vi "Insert Value (Nested String).vi"(7 "key":string[](array[string]), 8 "error in (no error)":errorcluster, 10 "JSON Data in":string, 11 "JSON Value in":refnum<class "JSON Value.lvclass">) -> (0 "error out":errorcluster, 1 "replaced":bool, 3 "JSON Value out":refnum<class "JSON Value.lvclass">)   [LabVIEW 2016, in "JSON Value.lvclass"]
uses:
  JSON Value.lvclass
  New JSON Value/New JSON String.vi
  Insert Value (Single).vi
  Array/Replace Array Subset/Replace Array Subset (Single).vi
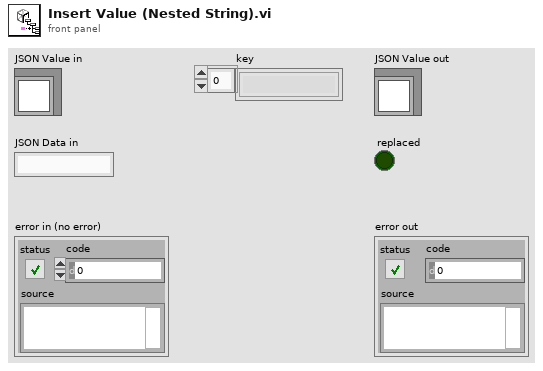
[diagram p1: front panel]
types:
  T1 = typedef "JSON Value.lvclass/JSON Types.ctl" = enum16{"String", "Numeric", "Boolean", "NULL", "Object", "Array"}
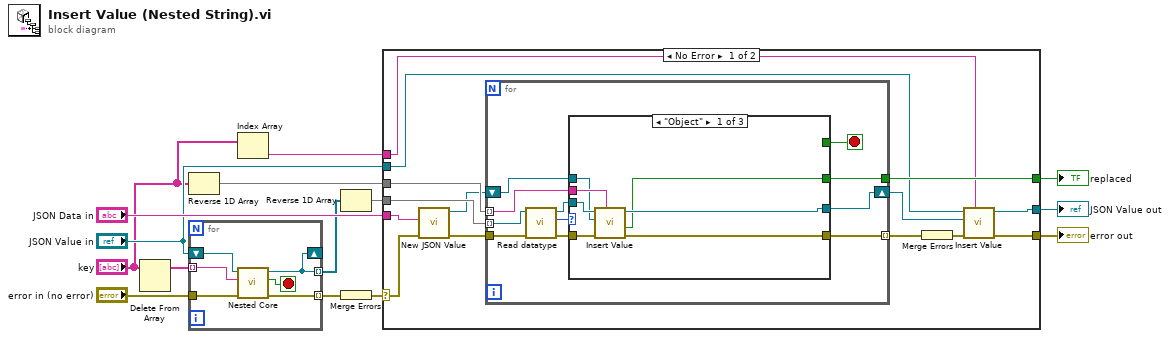
[diagram p0: block diagram]
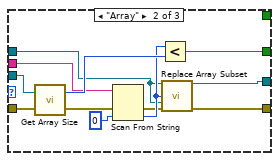
[diagram p2: hidden frame]
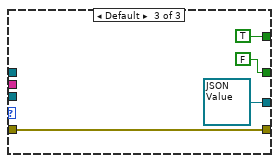
[diagram p3: hidden frame]
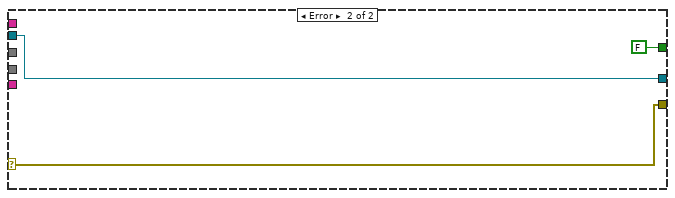
[diagram p4: hidden frame]
diagram:
  n1 = Delete From Array(array="key") -> (array with subset deleted=w10:string[])  [unwired: 2 in, 1 out]
  n2 = Reverse 1D Array(array="key") -> (reversed array=w11:string[])
  n3 = for {
    tunnel: w10 -> [w20] mode=indexing
    shift-right: [w15] -> _
    shift-left: "JSON Value in" -> [w19]
    tunnel: "error in (no error)" -> [w18]
    tunnel: [w17] -> w7 mode=indexing
    tunnel: [w15] -> w8 mode=indexing
    stop <- w16 stop-if-true
    n4 = call "Nested Core.vi"("error in (no error)"=w18, "key"=w20, "JSON Value in"=w19) -> ("error out"=w17:errorcluster, "stop?"=w16:bool, "JSON Value out"=w15:refnum<class "JSON Value.lvclass">)  [unwired: 6 in]
  }
  n5 = Index Array(array="key") -> (element=w1:string)  [unwired: 1 in]
  n6 = Reverse 1D Array(array=w8) -> (reversed array=w12:refnum<class "JSON Value.lvclass">[])
  n7 = Merge Errors(w7) -> (w9:errorcluster)
  n8 = case shown="No Error" w9 {
    selector: w9 -> [w22 w69]
    tunnel: [w34 FALSE ("replaced")] -> w14
    tunnel: "JSON Data in" -> [w24 _]
    tunnel: w12 -> [w33 _]
    tunnel: w11 -> [w32 _]
    tunnel: [w28 w71] -> w4
    tunnel: "JSON Value in" -> [w30 w71]
    tunnel: [w26 w69] -> w3
    tunnel: w1 -> [w25 _]
    frame No Error {
      n9 = call-poly "New JSON Value.vi"("error in (no error)"=w22, "value"=w24) -> ("error out"=w21:errorcluster, "JSON Value out"=w23:refnum<class "JSON Value.lvclass">)  [unwired: 8 in]
      n10 = for {
        tunnel: w32 -> [w37] mode=indexing
        tunnel: w21 -> [w43]
        tunnel: [w42] -> w31 mode=indexing
        tunnel: [w39] -> w34
        tunnel: w33 -> [w38] mode=indexing
        shift-right: [w36] -> w29
        shift-left: w23 -> [w35]
        stop <- w40 stop-if-true
        n11 = call "Read datatype.vi"("error in (no error)"=w43, "JSON Datatype in"=w38) -> ("error out"=w41:errorcluster, "datatype"=w44:T1, "JSON Datatype out"=w45:refnum<class "JSON Value.lvclass">)  [unwired: 7 in]
        n12 = case shown="\"Object\"" w44 {
          tunnel: w37 -> [w49 w61 _]
          tunnel: [w51 w59 refnum<class "JSON Value.lvclass"> refnum ("JSON Array")] -> w36
          tunnel: w45 -> [w48 w60 _]
          tunnel: [w52 w53 w67] -> w42
          tunnel: w41 -> [w47 w56 w67]
          tunnel: [_ _ TRUE] -> w40
          tunnel: [w50 w62 FALSE] -> w39
          tunnel: w35 -> [w46 w57 _]
          frame "Object" {
            n13 = call-poly "Insert Value.vi"("key"=w49, "error in (no error)"=w47, 10:"JSON Value in"=w46, 11:"JSON Value in"=w48) -> ("error out"=w52:errorcluster, "replaced"=w50:bool, "JSON Value out"=w51:refnum<class "JSON Value.lvclass">)  [unwired: 5 in]
          }
          frame "Array" {
            n14 = call "Get Array Size.vi"("error in (no error)"=w56, "JSON Value in"=w60) -> ("error out"=w55:errorcluster, "size(s)"=w63:i32)
            n15 = Scan From String(input string=w61, error in=w55, default 1=0 ("index")) -> (error out=w54:errorcluster, output 1=w58:i32)  [unwired: 2 in, 2 out]
            n16 = Less?(x=w58, y=w63) -> (x < y?=w62:bool)
            n17 = call-poly "Replace Array Subset.vi"("JSON Array"=w57, "index"=w58, "new element/subarray"=w57, "error in"=w54) -> ("output JSON Array"=w59:refnum<class "JSON Value.lvclass">, "error out"=w53:errorcluster)  [unwired: 10 in]
          }
          frame Default {
          }
        }
      }
      n18 = Merge Errors(w31) -> (w27:errorcluster)
      n19 = call-poly "Insert Value.vi"("key"=w25, "error in (no error)"=w27, 10:"JSON Value in"=w29, 11:"JSON Value in"=w30) -> ("error out"=w26:errorcluster, "JSON Value out"=w28:refnum<class "JSON Value.lvclass">)  [unwired: 5 in, 1 out]
    }
    frame Error {
    }
  }
  "replaced" <- w14
  "error out" <- w3
  "JSON Value out" <- w4
